vi "Angle to PWM middle(SubVI).vi"(11 "Angle in degrees":dbl) -> ()   [LabVIEW 2016]
uses:
  <vilib>/myRIO/Instrument Drivers/Onboard IO/PWM/typedefs/PWM Reference.ctl
  <vilib>/myRIO/Common/Instrument Driver Framework/Utilities/typedefs/myRIO Generic Hardware Reference.ctl
  <vilib>/myRIO/Common/Instrument Driver Framework/Utilities/typedefs/Hardware Version Enum.ctl
  <vilib>/myRIO/Common/Instrument Driver Framework/Utilities/typedefs/myRIO v1.0 Reference.ctl
  <vilib>/myRIO/Common/Instrument Driver Framework/Utilities/typedefs/Generic FPGA Reference.ctl
  <vilib>/myRIO/Common/Instrument Driver Framework/myRIO v1.0/PWM/typedefs/PWM Channels Enum.ctl
  <vilib>/myRIO/Instrument Drivers/Onboard IO/PWM/typedefs/PWM Configuration.ctl
  <vilib>/userdefined/High Color/nirio_resource_hc.ctl
  <vilib>/myRIO/Common/Instrument Driver Framework/Utilities/vis/Is FPGA Ref Available.vi
  <vilib>/myRIO/Common/Instrument Driver Framework/roboRIO v1.0/PWM/vis/roboRIO v1.0 Open PWM.vi
  <vilib>/myRIO/Instrument Drivers/Onboard IO/PWM/vis/Set Duty Cycle and Frequency.vi
  <vilib>/myRIO/Common/Instrument Driver Framework/Utilities/vis/Validate Channels.vi
  <vilib>/myRIO/Common/Instrument Driver Framework/roboRIO v1.0/PWM/vis/roboRIO v1.0 Reserve PWM.vi
  <vilib>/myRIO/Common/Instrument Driver Framework/roboRIO v1.0/PWM/vis/roboRIO v1.0 Build MUX Configuration PWM.vi
  <vilib>/myRIO/Common/Instrument Driver Framework/roboRIO v1.0/Resource Manager/vis/roboRIO v1.0 Reserve Channel List.vi
  <vilib>/myRIO/Common/Instrument Driver Framework/roboRIO v1.0/Resource Manager/vis/roboRIO v1.0 Create Configuration List.vi
  <vilib>/myRIO/Common/Instrument Driver Framework/roboRIO v1.0/Resource Manager/vis/roboRIO v1.0 Reserve Channel.vi
  <vilib>/myRIO/Common/Instrument Driver Framework/roboRIO v1.0/Resource Manager/vis/roboRIO v1.0 Unreserve Channel.vi
  <vilib>/myRIO/Common/Instrument Driver Framework/roboRIO v1.0/Resource Manager/vis/roboRIO v1.0 Build Mutex Name.vi
  <vilib>/Utility/VariantDataType/GetNumericInfo.vi
  <vilib>/Utility/error.llb/Error Cluster From Error Code.vi
  <vilib>/myRIO/Common/Instrument Driver Framework/roboRIO v1.0/roboRIO v1.0 Open.vi
  <vilib>/myRIO/Common/Instrument Driver Framework/Utilities/vis/IO Manager.vi
  <vilib>/myRIO/Common/Instrument Driver Framework/Utilities/vis/Configuration Manager.vi
  <vilib>/myRIO/Common/Instrument Driver Framework/roboRIO v1.0/Resource Manager/vis/roboRIO v1.0 Configure IO.vi
  <vilib>/myRIO/Common/Instrument Driver Framework/myRIO v1.0/myRIO v1.0 Close.vi
  <vilib>/myRIO/Common/Instrument Driver Framework/roboRIO v1.0/PWM/vis/roboRIO v1.0 Write PWM.vi
  <vilib>/myRIO/Express VI/Onboard IO/PWM/PWM Express VI.xnode
  <vilib>/myRIO/Instrument Drivers/Onboard IO/PWM/vis/myRIO PWM Open.xnode
  <vilib>/myRIO/Instrument Drivers/Onboard IO/PWM/PWM.lvlib
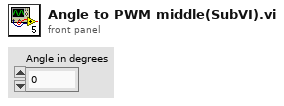
[diagram p1: front panel]
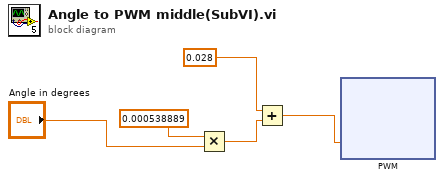
[diagram p0: block diagram]
diagram:
  n1 = Multiply(x=0.000538889, y="Angle in degrees") -> (x*y=w5:dbl)
  n2 = Add(x=0.028, y=w5) -> (x+y=w2:dbl)
  n3 = xnode "PWM"("Duty Cycle"=w2) -> ()  [unwired: 1 in, 1 out]
